vi "Post-Uninstall Custom Action.vi"(10 "Variant":variant) -> (0 "error out":errorcluster)   [LabVIEW 2017]
uses:
  <userlib>/NEVSTOP-Programming-Palette/Dialog & Interface/Fit VI window to Largest Dec_nevstop.vi
panel:
  in  "introduction 3":string="Click button to reset LabVIEW as the default option for LabVIEW file formats."
  in  "Reset Registry":bool
  out "dup file":path
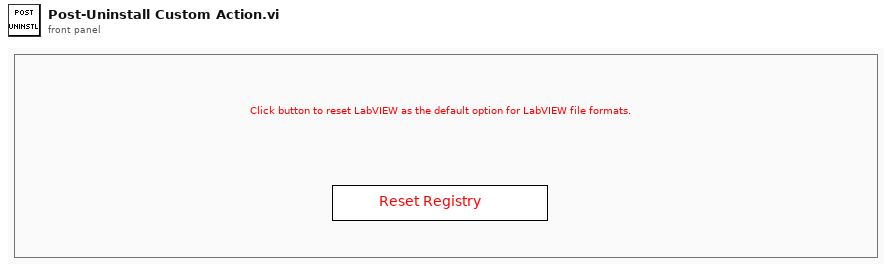
[diagram p1: front panel]
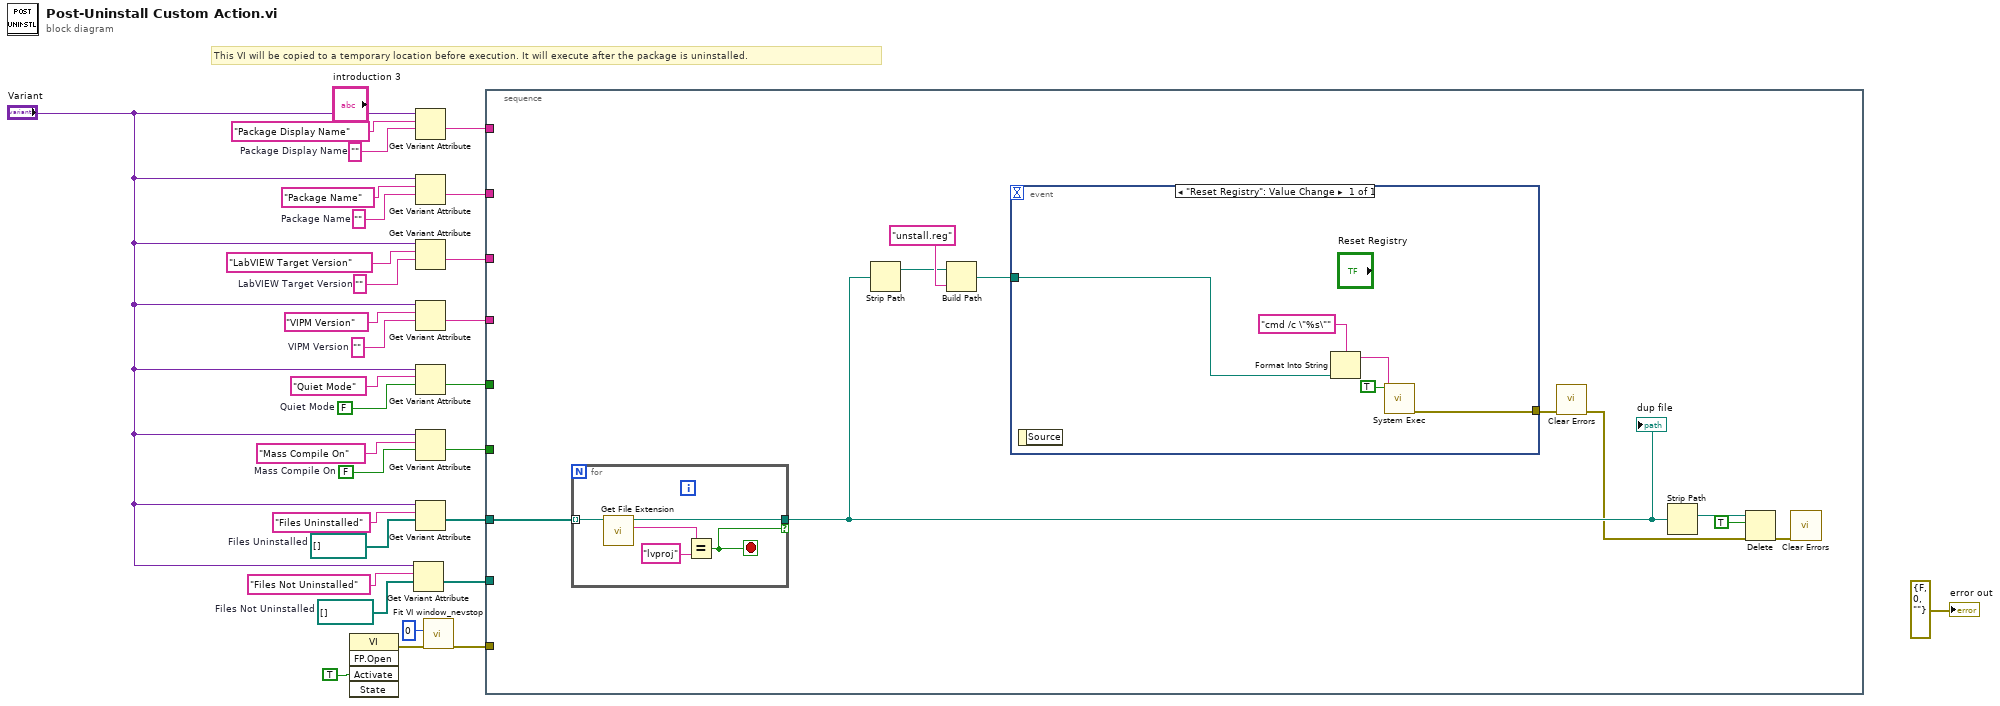
[diagram p0: block diagram]
diagram:
  w5 = path[] []  # Files Not Uninstalled
  w6 = path[] []  # Files Uninstalled
  w12 = FALSE  # Mass Compile On
  w13 = ""  # Package Display Name
  w20 = FALSE  # Quiet Mode
  w23 = ""  # VIPM Version
  w25 = ""  # LabVIEW Target Version
  w27 = ""  # Package Name
  # "This VI will be copied to a temporary location before execution. It will execute after the package is uninstalled."
  n1 = invoke class="VI" method="FP.Open"("Activate"=TRUE ("Activate?")) -> (error out=w2:errorcluster)  [unwired: 4 in, 4 out]
  n2 = Get Variant Attribute(Variant="Variant", name="Files Not Uninstalled", default value (empty Variant)=w5) -> (value=w10:path[])  [unwired: 1 in, 3 out]
  n3 = Get Variant Attribute(Variant="Variant", name="Package Display Name", default value (empty Variant)=w13) -> (value=w19:string)  [unwired: 1 in, 3 out]
  n4 = Get Variant Attribute(Variant="Variant", name="Package Name", default value (empty Variant)=w27) -> (value=w18:string)  [unwired: 1 in, 3 out]
  n5 = Get Variant Attribute(Variant="Variant", name="LabVIEW Target Version", default value (empty Variant)=w25) -> (value=w17:string)  [unwired: 1 in, 3 out]
  n6 = Get Variant Attribute(Variant="Variant", name="VIPM Version", default value (empty Variant)=w23) -> (value=w16:string)  [unwired: 1 in, 3 out]
  n7 = Get Variant Attribute(Variant="Variant", name="Quiet Mode", default value (empty Variant)=w20) -> (value=w15:bool)  [unwired: 1 in, 3 out]
  n8 = Get Variant Attribute(Variant="Variant", name="Mass Compile On", default value (empty Variant)=w12) -> (value=w14:bool)  [unwired: 1 in, 3 out]
  n9 = Get Variant Attribute(Variant="Variant", name="Files Uninstalled", default value (empty Variant)=w6) -> (value=w9:path[])  [unwired: 1 in, 3 out]
  n10 = call-poly <userlib>:"Fit VI window_nevstop.vi"("error in (no error)"=w2, "border spacing (2 px)"=0) -> ("error out"=w4:errorcluster)  [unwired: 4 in, 1 out]
  n11 = stacked-sequence {
    tunnel: w19 -> [_]
    tunnel: w18 -> [_]
    tunnel: w17 -> [_]
    tunnel: w16 -> [_]
    tunnel: w15 -> [_]
    tunnel: w14 -> [_]
    tunnel: w9 -> [w40]
    tunnel: w10 -> [_]
    tunnel: w4 -> [_]
    frame #0 {
      n12 = for {
        tunnel: w40 -> [w50] mode=indexing
        tunnel: [w49] -> w34 if=w47
        stop <- w47 stop-if-true
        n13 = call <vilib>:"Get File Extension.vi"("file"=w50) -> ("lowercase file extension"=w46:string, "dup file"=w49:path)  [unwired: 6 in, 3 out]
        n14 = Equal?(x=w46, y="lvproj") -> (x = y?=w47:bool)
      }
      "dup file" <- w34
      n15 = Strip Path(path=w34) -> (stripped path=w33:path)  [unwired: 1 out]
      n16 = Build Path(base path=w33, name or relative path="unstall.reg") -> (appended path=w35:path)
      n17 = event shown="[0] \"Reset Registry\": Value Change" {
        selector: _ -> [_]
        dyn-events: _ -> [_]
        timeout: _ -> [_]
        tunnel: w35 -> [w41]
        tunnel: [w42] -> w32
        event "Reset Registry": Value Change {
          n18 = event-data() -> ()  [unwired: 1 in, 1 out]
          n19 = Format Into String(format string="cmd /c \"%s\"", w41) -> (resulting string=w45:string)  [unwired: 2 in, 1 out]
          n20 = call <vilib>:"System Exec.vi"("run minimized? (F)"=TRUE, "command line"=w45) -> ("error out"=w42:errorcluster)  [unwired: 6 in, 3 out]
        }
      }
      n21 = call <vilib>:"Clear Errors.vi"("error in (no error)"=w32) -> ("error out"=w31:errorcluster)  [unwired: 5 in, 1 out]
      n22 = Strip Path(path=w34) -> (stripped path=w39:path)  [unwired: 1 out]
      n23 = Delete(path (use dialog)=w39, entire hierarchy (F)=TRUE, error in=w31) -> (error out=w37:errorcluster)  [unwired: 2 in, 2 out]
      n24 = call <vilib>:"Clear Errors.vi"("error in (no error)"=w37) -> ()  [unwired: 5 in, 2 out]
    }
  }
  "error out" <- errorcluster {"status"=FALSE, "code"=0, "source"=""} ("error out")
